vi "CopyDerivedNodes.vi"(6 "non device channels":string[](array[string]), 9 "parent channel":T1, 10 "channels in":T1[](array[typedef]), 11 "child nodes":T4[](array[typedef])) -> (2 "channels out":T1[](array[typedef]))   [LabVIEW 2017, in "ServerComm.lvlib"]
uses:
  <vilib>/addons/InsightCM/Devices/Shared/Common/ServerComm/ServerComm.lvlib
  <vilib>/addons/InsightCM/MessageBus/Base/controls/AssetNode.ctl
  <vilib>/addons/InsightCM/MessageBus/Base/controls/AssetState.ctl
  <vilib>/addons/InsightCM/MessageBus/Base/controls/KeyValuePair.ctl
  <vilib>/addons/InsightCM/MessageBus/Base/controls/OperatingState.ctl
  <vilib>/addons/InsightCM/MessageBus/Base/controls/Trigger.ctl
  <vilib>/addons/InsightCM/MessageBus/Base/controls/Condition.ctl
  <vilib>/addons/InsightCM/MessageBus/Base/controls/Metric.ctl
  <vilib>/addons/InsightCM/MessageBus/Base/controls/TrendAlarmRule.ctl
  <vilib>/addons/InsightCM/MessageBus/Base/controls/TrendAlarmLevel.ctl
  <vilib>/addons/InsightCM/MessageBus/Base/controls/AlarmAction.ctl
  <vilib>/addons/InsightCM/MessageBus/Base/controls/AssetNodeReference.ctl
  <vilib>/addons/InsightCM/MessageBus/Base/controls/R2_Channel.ctl
  <vilib>/addons/InsightCM/Utilities/PropertyHelpers/PropertyHelpers.lvlib
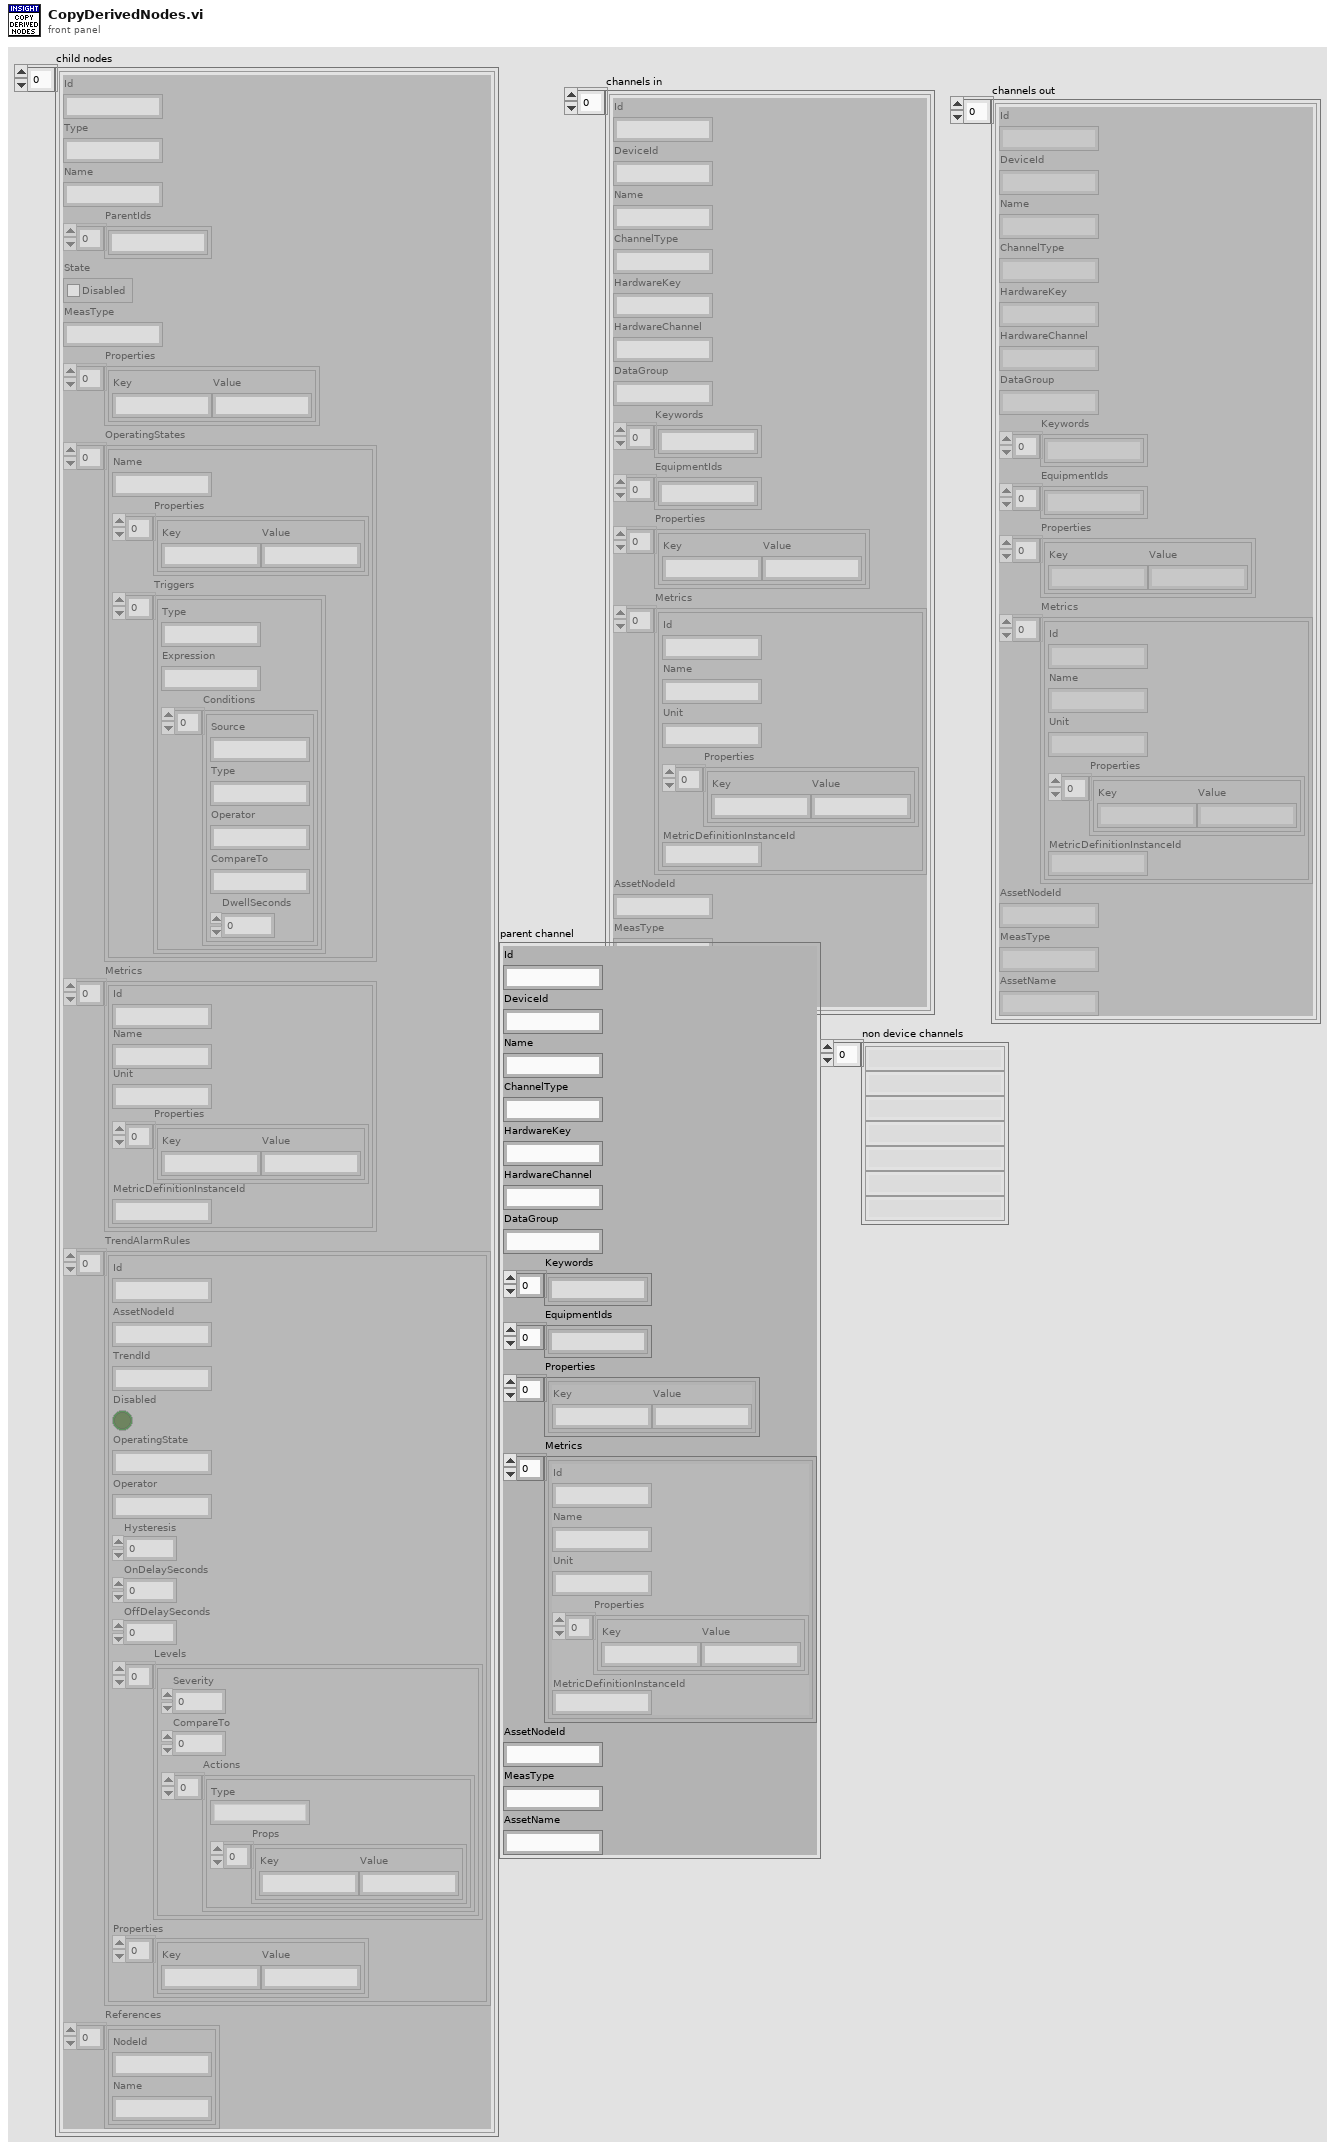
[diagram p1: front panel]
types:
  T1 = typedef "R2_Channel.ctl" = cluster{"Id":string, "DeviceId":string, "Name":string, "ChannelType":string, "HardwareKey":string, "HardwareChannel":string, "DataGroup":string, "Keywords":string[], "EquipmentIds":string[], "Properties":T2[], "Metrics":T3[], "AssetNodeId":string, "MeasType":string, "AssetName":string}
  T2 = typedef "KeyValuePair.ctl" = cluster{"Key":string, "Value":string}
  T3 = typedef "Metric.ctl" = cluster{"Id":string, "Name":string, "Unit":string, "Properties":T2[], "MetricDefinitionInstanceId":string}
  T4 = typedef "AssetNode.ctl" = cluster{"Id":string, "Type":string, "Name":string, "ParentIds":string[], "State":T5, "MeasType":string, "Properties":T2[], "OperatingStates":T6[], "Metrics":T3[], "TrendAlarmRules":T9[], "References":T12[]}
  T5 = typedef "AssetState.ctl" = cluster{"Disabled":bool}
  T6 = typedef "OperatingState.ctl" = cluster{"Name":string, "Properties":T2[], "Triggers":T7[]}
  T7 = typedef "Trigger.ctl" = cluster{"Type":string, "Expression":string, "Conditions":T8[]}
  T8 = typedef "Condition.ctl" = cluster{"Source":string, "Type":string, "Operator":string, "CompareTo":string, "DwellSeconds":dbl}
  T9 = typedef "TrendAlarmRule.ctl" = cluster{"Id":string, "AssetNodeId":string, "TrendId":string, "Disabled":bool, "OperatingState":string, "Operator":string, "Hysteresis":dbl, "OnDelaySeconds":dbl, "OffDelaySeconds":dbl, "Levels":T10[], "Properties":T2[]}
  T10 = typedef "TrendAlarmLevel.ctl" = cluster{"Severity":i32, "CompareTo":dbl, "Actions":T11[]}
  T11 = typedef "AlarmAction.ctl" = cluster{"Type":string, "Props":T2[]}
  T12 = typedef "AssetNodeReference.ctl" = cluster{"NodeId":string, "Name":string}
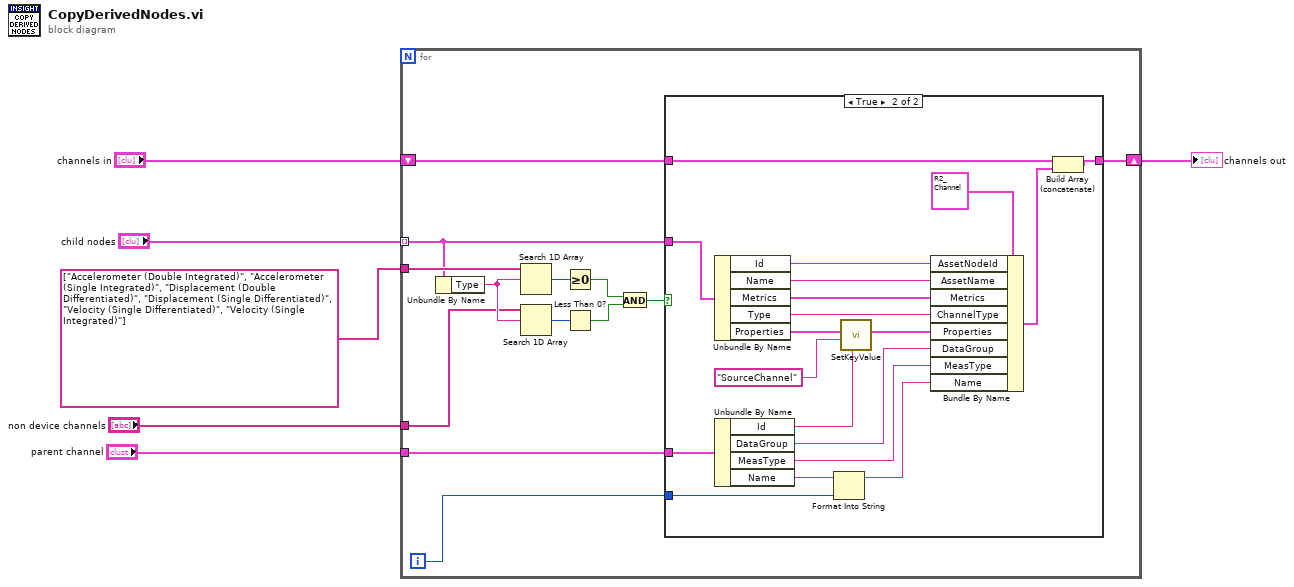
[diagram p0: block diagram]
diagram:
  n1 = for {
    tunnel: "child nodes" -> [w17] mode=indexing
    tunnel: string[] ["Accelerometer (Double Integrated)", "Accelerometer (Single Integrated)", "Displacement (Double Differentiated)", "Displacement (Single Differentiated)", "Velocity (Single Differentiated)", "Velocity (Single Integrated)"] ("Array") -> [w19]
    shift-right: [w16] -> w3
    shift-left: "channels in" -> [w18]
    tunnel: "parent channel" -> [w15]
    tunnel: "non device channels" -> [w9]
    i -> [w14]
    n2 = Unbundle By Name(w17) -> ("Type"=w10:string)
    n3 = Search 1D Array(1D array=w19, element=w10) -> (index of element=w13:i32)  [unwired: 1 in]
    n4 = Search 1D Array(1D array=w9, element=w10) -> (index of element=w8:i32)  [unwired: 1 in]
    n5 = Greater Or Equal To 0?(x=w13) -> (x >= 0?=w12:bool)
    n6 = Less Than 0?(x=w8) -> (x < 0?=w7:bool)
    n7 = And(x=w12, y=w7) -> (x .and. y?=w11:bool)
    n8 = case shown="True" w11 {
      tunnel: w18 -> [w20 w39]
      tunnel: w17 -> [_ w37]
      tunnel: [w20 w33] -> w16
      tunnel: w15 -> [_ w31]
      tunnel: w14 -> [_ w22]
      frame False {
      }
      frame True {
        n9 = Unbundle By Name(w37) -> ("Id"=w24:string, "Name"=w36:string, "Metrics"=w35:T3[], "Type"=w32:string, "Properties"=w29:T2[])
        n10 = Unbundle By Name(w31) -> ("Id"=w26:string, "DataGroup"=w30:string, "MeasType"=w25:string, "Name"=w23:string)
        n11 = Format Into String(initial string=w23, w22) -> (resulting string=w21:string)  [unwired: 2 in, 1 out]
        n12 = call <vilib>:"SetKeyValue.vi"("value"=w26, "key"="SourceChannel", "key value pairs"=w29) -> ("key value pairs out"=w28:T2[])  [unwired: 8 in]
        n13 = Bundle By Name(cluster=T1 {"Id"="", "DeviceId"="", "Name"="", "ChannelType"="", "HardwareKey"="", "HardwareChannel"="", "DataGroup"="", "Keywords"=[], "EquipmentIds"=[], "Properties"=[], "Metrics"=[], "AssetNodeId"="", "MeasType"="", "AssetName"=""} ("ChannelModel"), "AssetNodeId"=w24, "AssetName"=w36, "Metrics"=w35, "ChannelType"=w32, "Properties"=w28, "DataGroup"=w30, "MeasType"=w25, "Name"=w21) -> (w34:T1)
        n14 = Build Array (concatenate)(w39, w34) -> (w33:T1[])
      }
    }
  }
  "channels out" <- w3
